vi "MMI_PEPS_2A7_Action.vi"(8 "error in":errorcluster caption="错误输入", 9 "Input2":T1, 10 "Input1":T2, 11 "PEPS":T3 {"任意门开启锁车报警" items=["无请求", "禁止", "启用", "预留"]; "天窗/遮阳帘关闭设置" items=["无请求", "天窗关闭", "遮阳帘关闭", "预留"]; "车窗透气开启设置" items=["无请求", "禁止", "启用", "预留"]; "前雨刮激活后雨刮" items=["无请求", "不激活", "激活", "预留"]; "AVM道路中标定请求" items=["无请求", "开始标定", "预留"]; "自动开关窗设置显示" items=["无请求", "RKE长按控制", "车钥匙控制", "预留"]; "迎宾灯功能开关" items=["无请求", "禁止", "启用", "预留"]; "钥匙忘车内锁车报警" items=["无请求", "禁止", "启用", "预留"]; "AVAS禁用设置" items=["无请求", "禁止", "启用", "预留"]; "电源非OFF锁车报警" items=["无请求", "禁止", "启用", "预留"]; "外后视镜倒车倾斜" items=["无请求", "禁止所有倾斜", "启用驾驶侧", "启用乘客侧", "启用所有侧"]}) -> (0 "error out":errorcluster caption="错误输出")   [LabVIEW 2013]
uses:
  MMI_PEPS_2A7.ctl
  SendCmdStr/Input1.ctl
  SendCmdStr/Input2.ctl
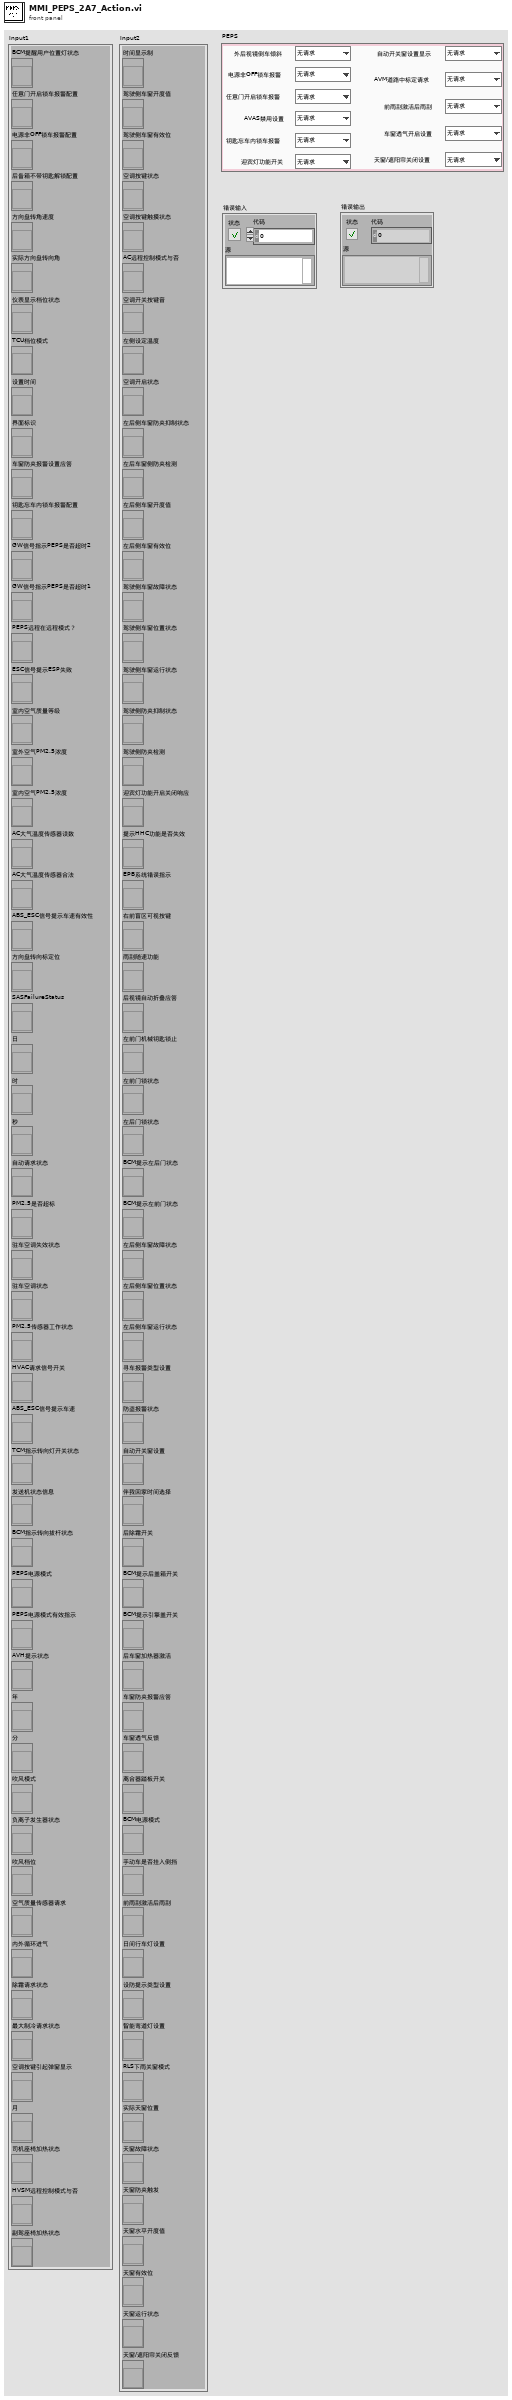
[diagram p1: front panel]
types:
  T1 = typedef "Input2.ctl" = cluster{"时间显示制":refnum<vi>, "驾驶侧车窗开度值":refnum<vi>, "驾驶侧车窗有效位":refnum<vi>, "空调按键状态":refnum<vi>, "空调按键触摸状态":refnum<vi>, "AC远程控制模式与否":refnum<vi>, "空调开关按键音":refnum<vi>, "左侧设定温度":refnum<vi>, "空调开启状态":refnum<vi>, "左后侧车窗防夹抑制状态":refnum<vi>, "左后车窗侧防夹检测":refnum<vi>, "左后侧车窗开度值":refnum<vi>, "左后侧车窗有效位":refnum<vi>, "驾驶侧车窗故障状态":refnum<vi>, "驾驶侧车窗位置状态":refnum<vi>, "驾驶侧车窗运行状态":refnum<vi>, "驾驶侧防夹抑制状态":refnum<vi>, "驾驶侧防夹检测":refnum<vi>, "迎宾灯功能开启关闭响应":refnum<vi>, "提示HHC功能是否失效":refnum<vi>, "EPB系统错误指示":refnum<vi>, "右前盲区可视按键":refnum<vi>, "雨刮随速功能":refnum<vi>, "后视镜自动折叠应答":refnum<vi>, "左前门机械钥匙锁止":refnum<vi>, "左前门锁状态":refnum<vi>, "左后门锁状态":refnum<vi>, "BCM提示左后门状态":refnum<vi>, "BCM提示左前门状态":refnum<vi>, "左后侧车窗故障状态":refnum<vi>, "左后侧车窗位置状态":refnum<vi>, "左后侧车窗运行状态":refnum<vi>, "寻车报警类型设置":refnum<vi>, "防盗报警状态":refnum<vi>, "自动开关窗设置":refnum<vi>, "伴我回家时间选择":refnum<vi>, "后除霜开关":refnum<vi>, "BCM提示后盖箱开关":refnum<vi>, "BCM提示引擎盖开关":refnum<vi>, "后车窗加热器激活":refnum<vi>, "车窗防夹报警应答":refnum<vi>, "车窗透气反馈":refnum<vi>, "离合器踏板开关":refnum<vi>, "BCM电源模式":refnum<vi>, "手动车是否挂入倒挡":refnum<vi>, "前雨刮激活后雨刮":refnum<vi>, "日间行车灯设置":refnum<vi>, "设防提示类型设置":refnum<vi>, "智能弯道灯设置":refnum<vi>, "RLS下雨关窗模式":refnum<vi>, "实际天窗位置":refnum<vi>, "天窗故障状态":refnum<vi>, "天窗防夹触发":refnum<vi>, "天窗水平开度值":refnum<vi>, "天窗有效位":refnum<vi>, "天窗运行状态":refnum<vi>, "天窗/遮阳帘关闭反馈":refnum<vi>}
  T2 = typedef "Input1.ctl" = cluster{"BCM提醒用户位置灯状态":refnum<vi>, "任意门开启锁车报警配置":refnum<vi>, "电源非OFF锁车报警配置":refnum<vi>, "后备箱不带钥匙解锁配置":refnum<vi>, "方向盘转角速度":refnum<vi>, "实际方向盘转向角":refnum<vi>, "仪表显示档位状态":refnum<vi>, "TCU档位模式":refnum<vi>, "设置时间":refnum<vi>, "界面标识":refnum<vi>, "车窗防夹报警设置应答":refnum<vi>, "钥匙忘车内锁车报警配置":refnum<vi>, "GW信号指示PEPS是否超时2":refnum<vi>, "GW信号指示PEPS是否超时1":refnum<vi>, "PEPS远程在远程模式？":refnum<vi>, "ESC信号提示ESP失败":refnum<vi>, "室内空气质量等级":refnum<vi>, "室外空气PM2.5浓度":refnum<vi>, "室内空气PM2.5浓度":refnum<vi>, "AC大气温度传感器读数":refnum<vi>, "AC大气温度传感器合法":refnum<vi>, "ABS_ESC信号提示车速有效性":refnum<vi>, "方向盘转向标定位":refnum<vi>, "SASFailureStatus":refnum<vi>, "日":refnum<vi>, "时":refnum<vi>, "秒":refnum<vi>, "自动请求状态":refnum<vi>, "PM2.5是否超标":refnum<vi>, "驻车空调失效状态":refnum<vi>, "驻车空调状态":refnum<vi>, "PM2.5传感器工作状态":refnum<vi>, "HVAC请求信号开关":refnum<vi>, "ABS_ESC信号提示车速":refnum<vi>, "TCM指示转向灯开关状态":refnum<vi>, "发送机状态信息":refnum<vi>, "BCM指示转向拔杆状态":refnum<vi>, "PEPS电源模式":refnum<vi>, "PEPS电源模式有效指示":refnum<vi>, "AVH提示状态":refnum<vi>, "年":refnum<vi>, "分":refnum<vi>, "吹风模式":refnum<vi>, "负离子发生器状态":refnum<vi>, "吹风档位":refnum<vi>, "空气质量传感器请求":refnum<vi>, "内外循环进气":refnum<vi>, "除霜请求状态":refnum<vi>, "最大制冷请求状态":refnum<vi>, "空调按键引起弹窗显示":refnum<vi>, "月":refnum<vi>, "司机座椅加热状态":refnum<vi>, "HVSM远程控制模式与否":refnum<vi>, "副驾座椅加热状态":refnum<vi>}
  T3 = typedef "MMI_PEPS_2A7.ctl" = cluster{"外后视镜倒车倾斜":u16, "电源非OFF锁车报警":u16, " 任意门开启锁车报警":u16, "AVAS禁用设置":u16, "钥匙忘车内锁车报警":u16, "迎宾灯功能开关":u16, "自动开关窗设置显示":u16, "AVM道路中标定请求":u16, "前雨刮激活后雨刮":u16, "车窗透气开启设置":u16, "天窗/遮阳帘关闭设置":u16}
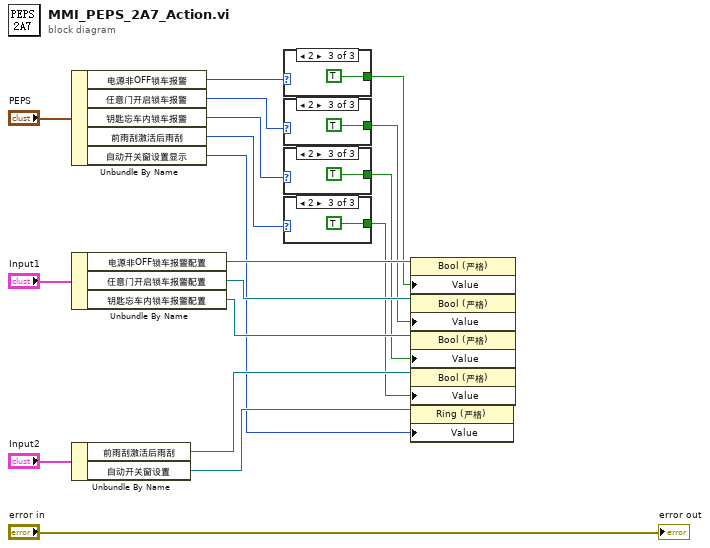
[diagram p0: block diagram]
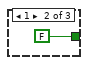
[diagram p3: hidden frame]
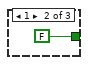
[diagram p5: hidden frame]
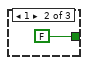
[diagram p7: hidden frame]
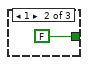
[diagram p9: hidden frame]
diagram:
  n1 = Unbundle By Name("PEPS") -> ("电源非OFF锁车报警"=w10:u16, "任意门开启锁车报警"=w8:u16, "钥匙忘车内锁车报警"=w6:u16, "前雨刮激活后雨刮"=w4:u16, "自动开关窗设置显示"=w2:u16)
  n2 = Unbundle By Name("Input1") -> ("电源非OFF锁车报警配置"=w15:refnum<vi>, "任意门开启锁车报警配置"=w14:refnum<vi>, "钥匙忘车内锁车报警配置"=w13:refnum<vi>)
  n3 = Unbundle By Name("Input2") -> ("前雨刮激活后雨刮"=w12:refnum<vi>, "自动开关窗设置"=w11:refnum<vi>)
  n4 = case shown="2" w10 {
    tunnel: [_ FALSE TRUE] -> w9
    frame 0, Default {
    }
    frame 1 {
    }
    frame 2 {
    }
  }
  n5 = case shown="2" w8 {
    tunnel: [_ FALSE TRUE] -> w7
    frame 0, Default {
    }
    frame 1 {
    }
    frame 2 {
    }
  }
  n6 = case shown="2" w6 {
    tunnel: [_ FALSE TRUE] -> w5
    frame 0, Default {
    }
    frame 1 {
    }
    frame 2 {
    }
  }
  n7 = case shown="2" w4 {
    tunnel: [_ FALSE TRUE] -> w3
    frame 0, Default {
    }
    frame 1 {
    }
    frame 2 {
    }
  }
  n8 = property class="Bool (严格)"(reference=w15, "Value"=w9) -> ()  [unwired: 1 in, 2 out]
  n9 = property class="Bool (严格)"(reference=w14, "Value"=w7) -> ()  [unwired: 1 in, 2 out]
  n10 = property class="Bool (严格)"(reference=w13, "Value"=w5) -> ()  [unwired: 1 in, 2 out]
  n11 = property class="Bool (严格)"(reference=w12, "Value"=w3) -> ()  [unwired: 1 in, 2 out]
  n12 = property class="Ring (严格)"(reference=w11, "Value"=w2) -> ()  [unwired: 1 in, 2 out]
  "error out" <- "error in"
